vi "Launch Report Viewer UI.vi"(8 "error in":errorcluster, 11 "Base Software in":refnum<class "Base Software.lvclass">) -> (0 "error out":errorcluster, 3 "Base Software out":refnum<class "Base Software.lvclass">)   [LabVIEW 2019, in "Base Software.lvlib" / "Main.lvlib" / "Base Software.lvclass"]
uses:
  Project/Base Software.lvclass
  C:/Users/Public/Documents/Development/builds/Engine/Engine.lvlibp/Project/Engine.lvclass
  builds/Engine/Panel Manager.lvlibp/Panel Actor/Panel Actor.lvclass
  builds/Engine/Panel.lvlibp/Panel/Panel.lvclass
  Custom Controls/Panel_Positions.ctl
  builds/Base Software/Panels/Report_Viewer.lvlibp/Library/Report Viewer.lvclass
  C:/Users/Public/Documents/Development/builds/Engine/Monitored Actor.lvlibp/Monitored Actor/Monitored Actor/Monitored Actor.lvclass
  C:/Users/Public/Documents/Development/builds/Engine/Panel Manager.lvlibp/Panel Actor/Panel Actor.lvclass
  builds/Engine/Panel.lvlibp/Panel/Subpanel/Subpanel.lvclass
  C:/Users/Public/Documents/Development/builds/Engine/Panel.lvlibp/Panel/Panel.lvclass
  builds/Engine/Engine.lvlibp/Accessors/Read Directory.vi
  builds/Engine/Engine.lvlibp/Accessors/Read Events.vi
  Accessors/GUI/Read Prime Panel ref.vi
  builds/Engine/Panel.lvlibp/Panel/Subpanel/Subpanel.vi
  Custom Controls/g_Identifiers.vi
  builds/Engine/Engine.lvlibp/Accessors/Write Directory.vi
  builds/Engine/Engine.lvlibp/Accessors/Write Events.vi
  builds/Engine/Panel.lvlibp
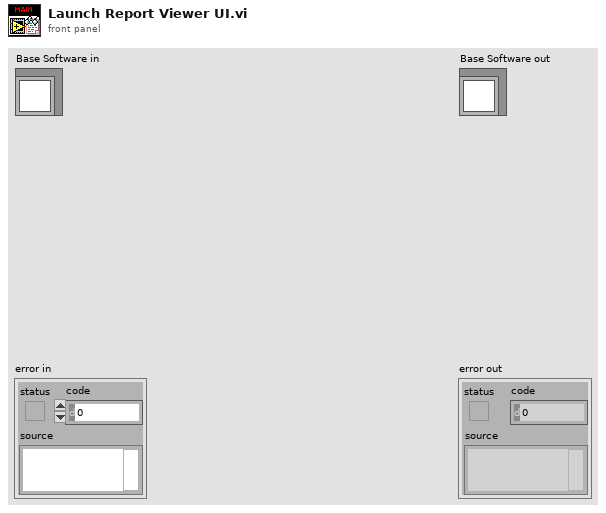
[diagram p1: front panel]
types:
  T1 = typedef "Base Software.lvlib/Main.lvlib/Base Software.lvclass/Panel_Positions.ctl" = enum16{"Prime", "Right", "Bottom", "Left", "Mission"}
  T2 = cluster{"Panel Actor":refnum<class "Panel Actor.lvclass">, "Panel":refnum<class "Panel.lvclass">}
  T3 = typedef "Engine.lvlibp/Engine.lvclass/Engine Events.ctl" = cluster{"System Event":T4, "Manual":T5, "UUT":T6, "Interface Events":T7}
  T4 = typedef "Engine.lvlibp/Engine.lvclass/System Events.ctl" = cluster{"Fault Event":refnum<user-event>, "SystemStatus Event":refnum<user-event>, "Automation":refnum<user-event>}
  T5 = typedef "Engine.lvlibp/Engine.lvclass/Manual Events.ctl" = cluster{"QuickStart Event":refnum<user-event>, "SafeBTE Event":refnum<user-event>, "TogglePower Event":refnum<user-event>, "Change Instrument Event":refnum<user-event>, "Toggle Launch Event":refnum<user-event>, "UUTSupply":refnum<user-event>}
  T6 = typedef "Engine.lvlibp/Engine.lvclass/UUT_Events.ctl" = cluster{"UUT_Name":refnum<user-event>, "Test_Name":refnum<user-event>, "Test_Operator":refnum<user-event>, "Test_Witness":refnum<user-event>, "Pedigree_Event":refnum<user-event>}
  T7 = typedef "Engine.lvlibp/Engine.lvclass/Interface Events.ctl" = cluster{"Interface_Command":refnum<user-event>, "Telemetry_Descriptor":refnum<user-event>, "AsynchTLM_Descriptor":refnum<user-event>}
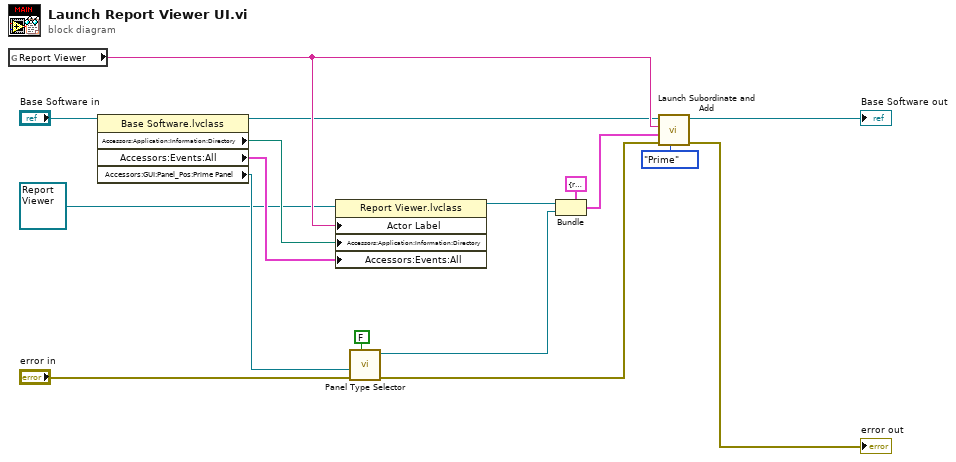
[diagram p0: block diagram]
diagram:
  n1 = global read "g_Identifiers.vi" "Report Viewer"() -> (w16:string)
  n2 = property class="Base Software.lvclass"(reference="Base Software in") -> (reference out=w5:refnum<class "Base Software.lvclass">, "Accessors:Application:Information:Directory"=w3:path, "Accessors:Events:All"=w4:T3, "Accessors:GUI:Panel_Pos:Prime Panel"=w6:refnum<vi>)  [unwired: 1 in, 1 out]
  n3 = property class="Report Viewer.lvclass"(reference=refnum<class "Report Viewer.lvclass"> refnum ("Report_Viewer.lvlibp:Report Viewer.lvclass"), "Actor Label"=w16, "Accessors:Application:Information:Directory"=w3, "Accessors:Events:All"=w4) -> (reference out=w15:refnum<class "Report Viewer.lvclass">)  [unwired: 1 in, 1 out]
  n4 = call-poly "Panel Type Selector.vi"("Autoshow? (T)"=FALSE, "Error In"="error in", "Sub Panel"=w6) -> ("Error Out"=w10:errorcluster, "Subpanel Out"=w12:refnum<class "Subpanel.lvclass">)  [unwired: 7 in]
  n5 = Bundle(cluster=T2 {"Panel Actor"=refnum, "Panel"=refnum} ("Panel Definiton"), "Panel Actor"=w15, "Panel"=w12) -> (w11:T2)
  n6 = call "Launch Subordinate and Add.vi"("Position"=Panel_Positions."Prime", "error in"=w10, "Panel Definiton"=w11, "Identifier"=w16, "Base Software in"=w5) -> ("error out"=→"error out":errorcluster, "Base Software out"=→"Base Software out":refnum<class "Base Software.lvclass">)  [unwired: 5 in]
